vi "Init.vi"(8 "error in":errorcluster) -> (0 "error out":errorcluster)   [LabVIEW 2009, in "Main.lvlib"]
doc: "Main initialization VI. Runs on the program startup."
uses:
  Main.lvlib
  CAN/SubVIs/CAN Jaguar Control Mode.ctl
  OWNCAN.lvlib
  FPGA.lvlib
  Servo.lvlib
  Utility.lvlib
  CAN.lvlib
  Drive.lvlib
  ImageProject/Camera.lvlib
  NetworkVarTarget.lvlib
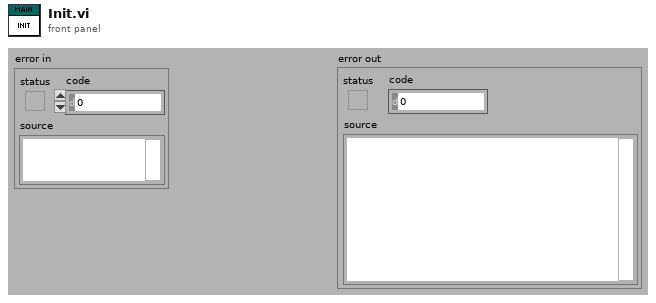
[diagram p1: front panel]
types:
  T1 = typedef "CAN.lvlib/CAN Jaguar Control Mode.ctl" = enum16{"Percent VBus", "Speed", "Position", "Current"}
  T2 = typedef "IMAQ Image.ctl" = refnum<image>
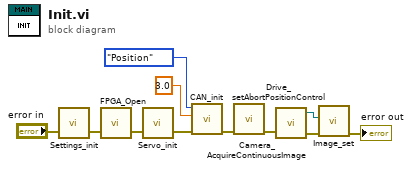
[diagram p0: block diagram]
diagram:
  n1 = call "Settings_init.vi"("error in"="error in") -> ("error out"=w11:errorcluster)  [unwired: 2 in]
  n2 = call "FPGA_Open.vi"("error in"=w11) -> ("error out"=w9:errorcluster)  [unwired: 2 in]
  n3 = call "Servo_init.vi"("error in (no error)"=w9) -> ("error out"=w8:errorcluster)  [unwired: 2 in]
  n4 = call "CAN_init.vi"("error in"=w8, "Maximum Output Voltage"=3.0, "Control Mode"=CAN_Jaguar_Control_Mode."Position") -> ("error out"=w5:errorcluster)  [unwired: 5 in, 1 out]
  n5 = call "Drive_setAbortPositionControl.vi"("error in (no error)"=w5) -> ("error out"=w4:errorcluster)  [unwired: 10 in]
  n6 = call "Camera_AcquireContinuousImage.vi"("error in"=w4) -> ("Image Out"=w1:T2, "error out"=w3:errorcluster)  [unwired: 1 in, 1 out]
  n7 = call "Image_set.vi"("error in (no error)"=w3, "Image"=w1) -> ("error out"=→"error out":errorcluster)  [unwired: 9 in]
